vi "Generate selector strings.vi"(9 "[POI#] or [MiniScan#]":T2 {"ROI number" min=1 format="ROI %.0f"}, 10 "POI Averaged":bool, 11 "Groups":T1[](array[typedef])) -> (1 "[Visibility]":bool[](array[boolean]), 3 "All group and ROI Strings[]":string[](array[string]))   [LabVIEW 2020]
uses:
  Typedefs/ROI selector array-ROI vis.ctl
  xcontrol/Interface VIs/Interface typedefs/Interface-ROI selection cluster.ctl
  Typedefs/ROI ID Enum.ctl
  Typedefs/Group sel cluster.ctl
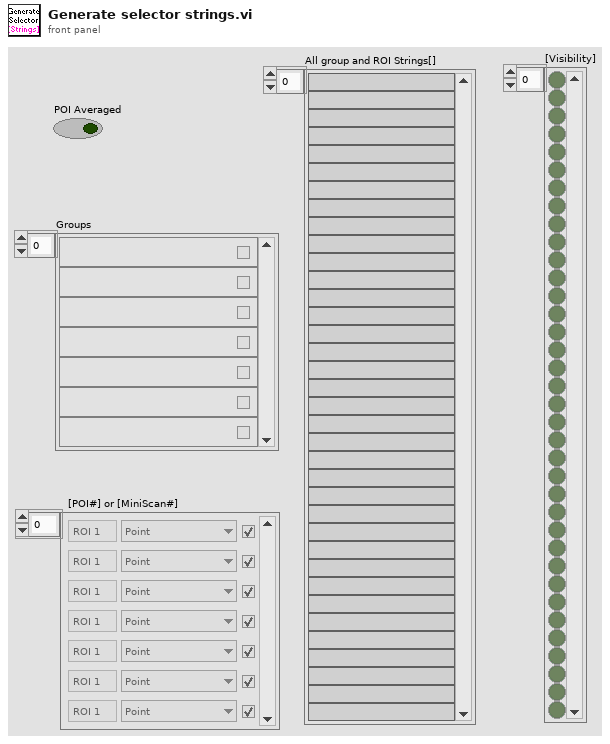
[diagram p1: front panel]
types:
  T1 = typedef "Group sel cluster.ctl" = cluster{"Group number":string, "Group Name":string, "Visibility":bool, "Highlight":bool}
  T2 = typedef "ROI selector array-ROI vis.ctl" = T3[]
  T3 = typedef "Interface-ROI selection cluster.ctl" = cluster{"ROI number":i32, "ROI ID":T4, "Visibility":bool}
  T4 = typedef "ROI ID Enum.ctl" = enum16{"Point", "MiniScan", "Comp. MiniScan", "Rectangle", "Comp. volume", "Arb. plane point", "None"}
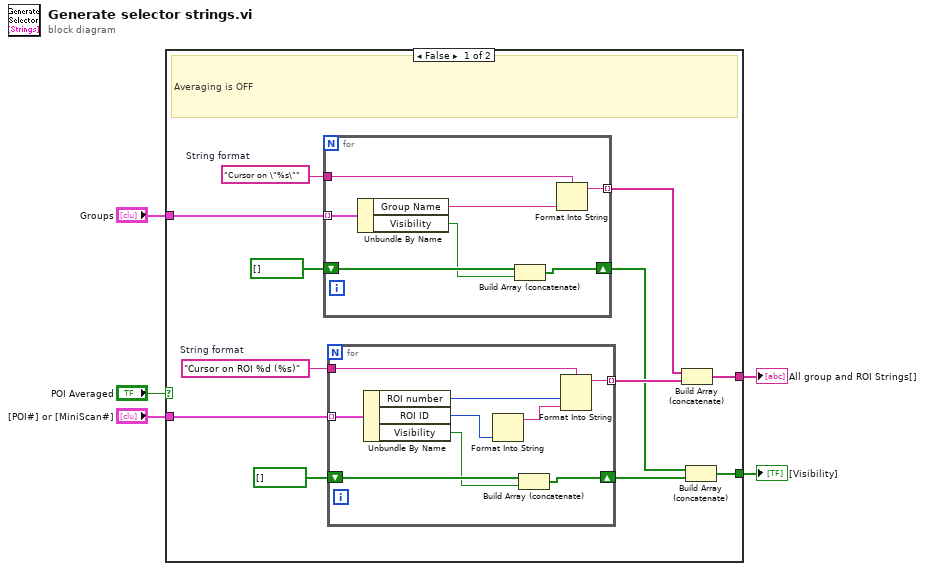
[diagram p0: block diagram]
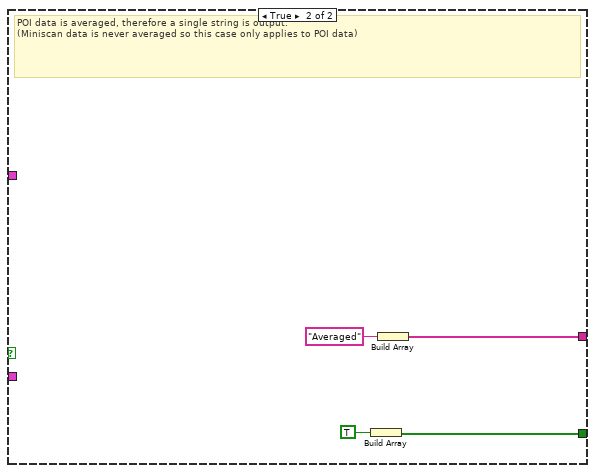
[diagram p2: hidden frame]
diagram:
  n1 = case shown="False" "POI Averaged" {
    tunnel: [w6 w34] -> w5
    tunnel: "[POI#] or [MiniScan#]" -> [w17 _]
    tunnel: [w11 w36] -> w3
    tunnel: "Groups" -> [w15 _]
    frame False {
      w14 = "Cursor on \"%s\""  # String format
      w16 = "Cursor on ROI %d (%s)"  # String format
      # "Averaging is OFF"
      n2 = for {
        tunnel: w15 -> [w22] mode=indexing
        tunnel: [w23] -> w9 mode=indexing
        tunnel: w14 -> [w24]
        shift-right: [w21] -> w8
        shift-left: bool[] [] -> [w20]
        n3 = Unbundle By Name(w22) -> ("Group Name"=w18:string, "Visibility"=w19:bool)
        n4 = Build Array (concatenate)(w20, w19) -> (w21:bool[])
        n5 = Format Into String(format string=w24, w18) -> (resulting string=w23:string)  [unwired: 2 in, 1 out]
      }
      n6 = for {
        tunnel: w17 -> [w31] mode=indexing
        tunnel: [w32] -> w10 mode=indexing
        tunnel: w16 -> [w33]
        shift-right: [w30] -> w7
        shift-left: bool[] [] -> [w29]
        n7 = Unbundle By Name(w31) -> ("ROI number"=w28:i32, "ROI ID"=w26:T4, "Visibility"=w27:bool)
        n8 = Format Into String(w26) -> (resulting string=w25:string)  [unwired: 3 in, 1 out]
        n9 = Build Array (concatenate)(w29, w27) -> (w30:bool[])
        n10 = Format Into String(format string=w33, w28, w25) -> (resulting string=w32:string)  [unwired: 2 in, 1 out]
      }
      n11 = Build Array (concatenate)(w9, w10) -> (w11:string[])
      n12 = Build Array (concatenate)(w8, w7) -> (w6:bool[])
    }
    frame True {
      # "POI data is averaged, therefore a single string is output.\n(Miniscan data is never averaged so this case only applies to POI data)"
      n13 = Build Array(TRUE) -> (w34:bool[])
      n14 = Build Array("Averaged") -> (w36:string[])
    }
  }
  "[Visibility]" <- w5
  "All group and ROI Strings[]" <- w3
